vi "Refname to String (Cameras).vi"(1 "Enum":T1) -> (0 "String":string)   [LabVIEW 2016]
uses:
  Cameras.ctl
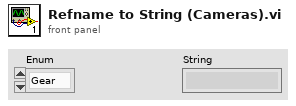
[diagram p1: front panel]
types:
  T1 = typedef "Cameras.ctl" = enum16{"Gear", "Climber"}
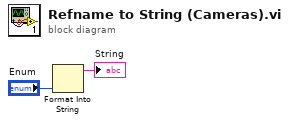
[diagram p0: block diagram]
diagram:
  n1 = Format Into String("Enum") -> (resulting string=→"String":string)  [unwired: 3 in, 1 out]
